vi "Start.Camera.vi"(8 "error in":errorcluster, 10 "Camera Address":string="cam0", 11 "CameraDevRef":T1={"Camera Address"="192.168.0.90", "CameraStatus"={"status"=FALSE, "code"=0, "source"=""}}) -> (0 "error out":errorcluster, 3 "CameraDevRef Out":T1)   [LabVIEW 2015]
uses:
  <vilib>/Rock Robotics/WPI/Camera/WPI_CameraImageSize.ctl
  <vilib>/Rock Robotics/WPI/Camera/WPI_CameraDevRef.ctl
  <vilib>/Rock Robotics/WPI/Camera/WPI_CameraWhite Balance Values.ctl
  <vilib>/Rock Robotics/WPI/Camera/WPI_CameraExposure Values.ctl
  <vilib>/Rock Robotics/WPI/Camera/WPI_CameraFrameRate.ctl
panel:
  in  "Image Size":T2=enum."320x240"
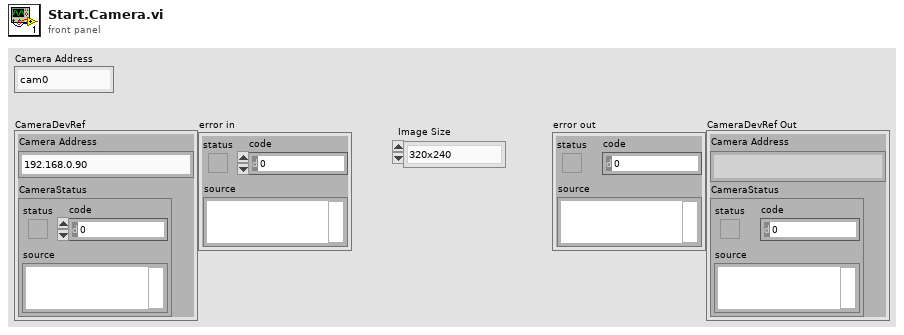
[diagram p1: front panel]
types:
  T1 = typedef "WPI_CameraDevRef.ctl" = cluster{"Camera Address":string, "CameraStatus":errorcluster}
  T2 = typedef "WPI_CameraImageSize.ctl" = enum16{"640x480", "320x240", "160x120", "Custom"}
  T3 = typedef "WPI_CameraFrameRate.ctl" = u32
  T4 = typedef "WPI_CameraExposure Values.ctl" = enum16{"Auto", "Flicker-free 50 Hz", "Flicker-free 60 Hz", "Hold current", "Custom"}
  T5 = typedef "WPI_CameraWhite Balance Values.ctl" = enum16{"Auto", "Fixed indoor", "Fixed outdoor 1", "Fixed outdoor 2", "Fixed fluorescent 1", "Fixed fluorescent 2", "Hold current", "Custom"}
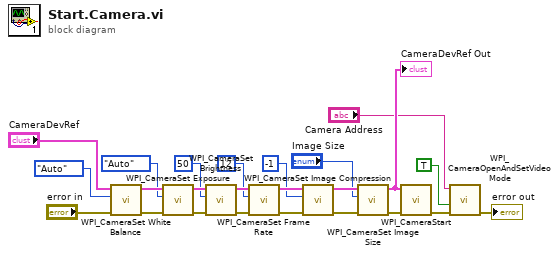
[diagram p0: block diagram]
diagram:
  n1 = call <vilib>:"WPI_CameraSet White Balance.vi"("error in (no error)"="error in", "White Balance"=WPI_CameraWhite_Balance_Values."Auto", "CameraDevRef"="CameraDevRef") -> ("error out"=w23:errorcluster, "CameraDevRef Out"=w24:T1)  [unwired: 1 in, 6 out]
  n2 = call <vilib>:"WPI_CameraSet Exposure.vi"("error in (no error)"=w23, "Exposure"=WPI_CameraExposure_Values."Auto", "CameraDevRef"=w24) -> ("error out"=w22:errorcluster, "CameraDevRef Out"=w21:T1)  [unwired: 1 in, 6 out]
  n3 = call <vilib>:"WPI_CameraSet Brightness.vi"("error in (no error)"=w22, "Brightness"=50, "CameraDevRef"=w21) -> ("error out"=w15:errorcluster, "CameraDevRef Out"=w16:T1)  [unwired: 7 out]
  n4 = call <vilib>:"WPI_CameraSet Frame Rate.vi"("error in (no error)"=w15, "Frame Rate (fps)"=T3 12, "CameraDevRef"=w16) -> ("error out"=w17:errorcluster, "CameraDevRef Out"=w20:T1)  [unwired: 7 out]
  n5 = call <vilib>:"WPI_CameraSet Image Compression.vi"("error in (no error)"=w17, "Compression"=-1, "CameraDevRef"=w20) -> ("error out"=w18:errorcluster, "CameraDevRef Out"=w19:T1)  [unwired: 7 out]
  n6 = call <vilib>:"WPI_CameraSet Image Size.vi"("error in (no error)"=w18, "Image Size"="Image Size", "CameraDevRef"=w19) -> ("error out"=w3:errorcluster, "CameraDevRef Out"=w4:T1)  [unwired: 1 in, 6 out]
  "CameraDevRef Out" <- w4
  n7 = call <vilib>:"WPI_CameraStart.vi"("error in (no error)"=w3, "CameraDevRef"=w4) -> ("error out"=w5:errorcluster)  [unwired: 8 in, 1 out]
  n8 = call <vilib>:"WPI_CameraOpenAndSetVideoMode.vi"("error in (no error)"=w5, "USB JPEG"=TRUE, "Camera Address Out"="Camera Address") -> ("error out"=→"error out":errorcluster)  [unwired: 8 in]
